vi "Quit.vi"(0 "Notifier Name":string, 11 "Error In":errorcluster) -> (4 "Notifier Name DUP":string, 15 "Error Out":errorcluster)   [LabVIEW 2020]
uses:
  Hardware Configuration/Hardware Configuration Controls/Company.ctl
  Hamamatsu/Orca Flash/Orca Flash Controls/Orca Flash Actions.ctl
  IDS/IDS Controls/IDS Actions.ctl
  Photometrics/Prime BSI/R Cubed SITK/Prime BSI R3 Controls/Prime R3 Actions.ctl
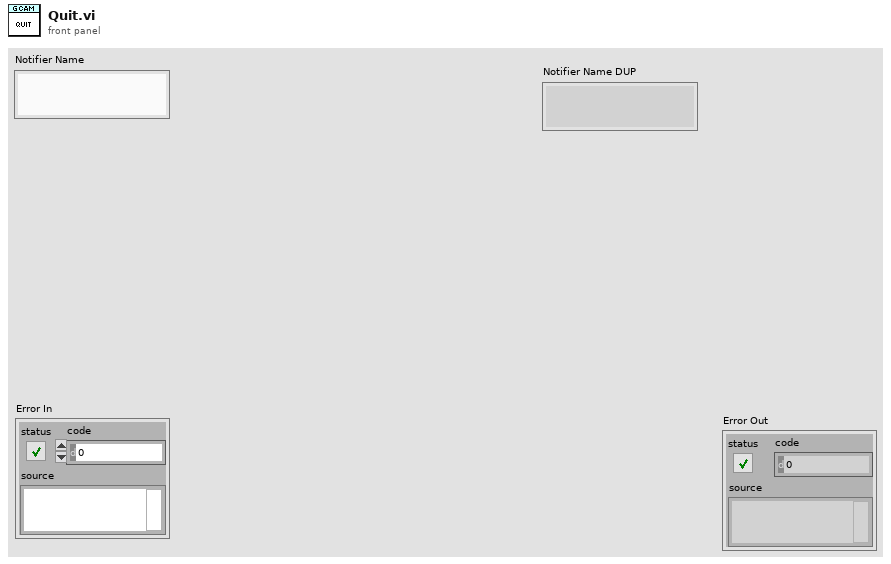
[diagram p1: front panel]
types:
  T1 = typedef "Company.ctl" = enum16{"AA Opto Electronic", "ASI", "Coherent", "Creset Optics", "CVI", "DAQmx", "Hamamatsu", "IDS", "Mad City Labs", "Marzhauser", "Measurement Computing", "MPB Com", "Olympus", "Photometrics", "PI", "Prior", "Thorlabs"}
  T2 = typedef "Orca Flash Actions.ctl" = enum16{"Idle", "Preview", "Record", "Record Settings", "Set Param", "Get Param", "Set ROI", "Get ROI", "Trigger Source", "Trigger Type", "Progessive Mode", "Area Mode", "Status", "Quit"}
  T3 = typedef "IDS Actions.ctl" = enum16{"Error Check", "Initialize", "Preview", "Record", "Abort", "Record Settings", "Set Parameter", "Get Parameter", "Set ROI", "Get ROI", "Status", "Quit"}
  T4 = typedef "Prime R3 Actions.ctl" = enum16{"Error Check", "Initialize", "Preview", "Record", "Abort", "Record Settings", "Set Parameter", "Get Parameter", "Set ROI", "Get ROI", "Status", "Set Trigger", "Quit"}
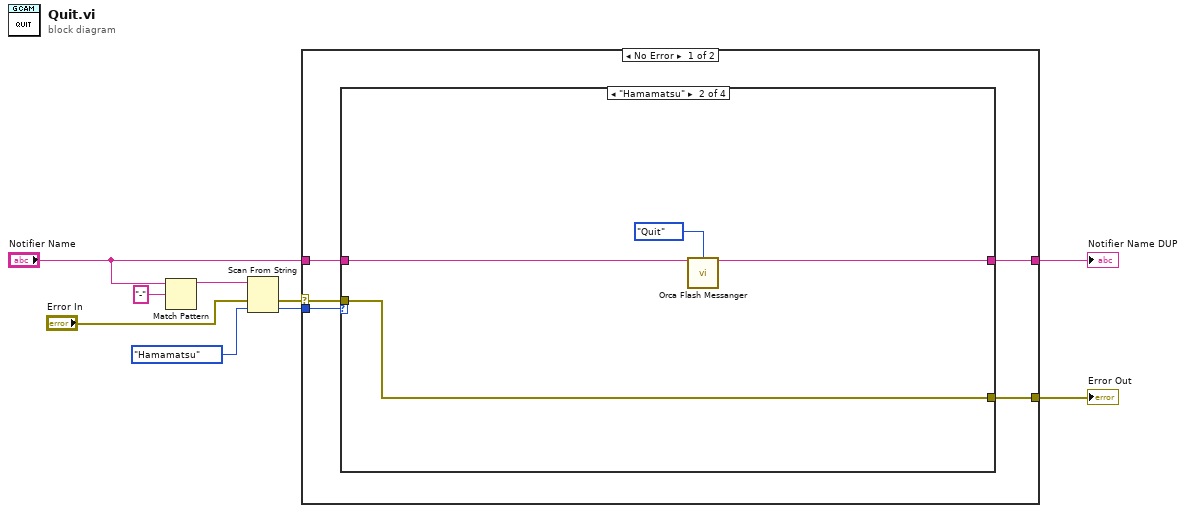
[diagram p0: block diagram]
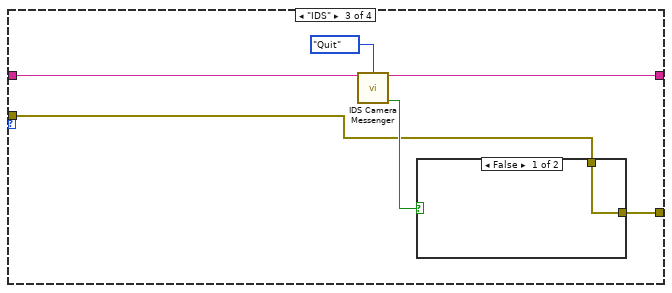
[diagram p3: hidden frame]
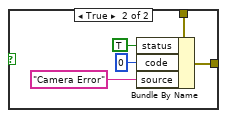
[diagram p4: hidden frame]
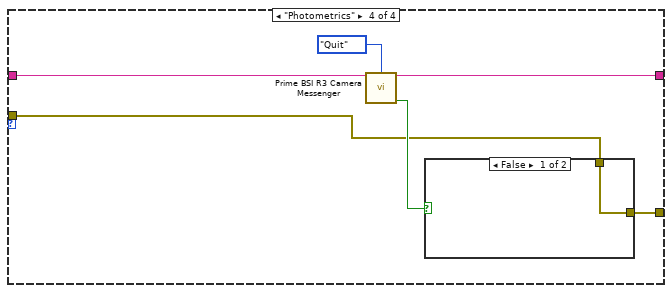
[diagram p5: hidden frame]
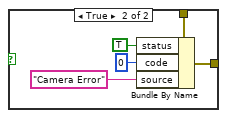
[diagram p6: hidden frame]
diagram:
  n1 = Match Pattern(string="Notifier Name", regular expression="-") -> (before substring=w7:string)  [unwired: 1 in, 3 out]
  n2 = Scan From String(input string=w7, error in="Error In", default 1=Company."Hamamatsu" ("Company")) -> (error out=w3:errorcluster, output 1=w6:T1)  [unwired: 2 in, 2 out]
  n3 = case shown="No Error" w3 {
    selector: w3 -> [w12 w45]
    tunnel: w6 -> [w14 _]
    tunnel: "Notifier Name" -> [w13 w46]
    tunnel: [w11 w46] -> w2
    tunnel: [w10 w45] -> w1
    frame No Error {
      n4 = case shown="\"Hamamatsu\"" w14 {
        tunnel: w13 -> [w16 w20 w26 w38]
        tunnel: w12 -> [w15 w18 w22 w35]
        tunnel: [w16 w19 w25 w37] -> w11
        tunnel: [w15 w18 w21 w34] -> w10
        frame Default {
        }
        frame "Hamamatsu" {
          n5 = call "Orca Flash Messanger.vi"("Notifier Name"=w20, "Camera Actions"=Orca_Flash_Actions."Quit") -> ("Notifier Name Dup"=w19:string)  [unwired: 9 in, 4 out]
        }
        frame "IDS" {
          n6 = call "IDS Camera Messenger.vi"("Notifier Name"=w26, "IDS Actions"=IDS_Actions."Quit") -> ("Notifier Name (Dup)"=w25:string, "Error?"=w23:bool)  [unwired: 8 in, 4 out]
          n7 = case shown="False" w23 {
            tunnel: w22 -> [w27 w32]
            tunnel: [w27 w31] -> w21
            frame False {
            }
            frame True {
              n8 = Bundle By Name(cluster=w32, "status"=TRUE, "code"=0, "source"="Camera Error") -> (w31:errorcluster)
            }
          }
        }
        frame "Photometrics" {
          n9 = call "Prime BSI R3 Camera Messenger.vi"("Notifier Name"=w38, "Prime Actions"=Prime_R3_Actions."Quit") -> ("Notifier Name (Dup)"=w37:string, "Error?"=w36:bool)  [unwired: 8 in, 4 out]
          n10 = case shown="False" w36 {
            tunnel: w35 -> [w39 w44]
            tunnel: [w39 w43] -> w34
            frame False {
            }
            frame True {
              n11 = Bundle By Name(cluster=w44, "status"=TRUE, "code"=0, "source"="Camera Error") -> (w43:errorcluster)
            }
          }
        }
      }
    }
    frame Error {
    }
  }
  "Error Out" <- w1
  "Notifier Name DUP" <- w2
